vi "MAIN_call.vi"(8 "error IN":errorcluster, 11 "VISA resource name out":refnum<visa-resource-name>) -> (0 "error out":errorcluster)   [LabVIEW 2019]
uses:
  VI's/ESTADOS_ABS.ctl
  <vilib>/Utility/error.llb/Error Cluster From Error Code.vi
  <vilib>/ErrorRing/Error Ring.xnode
  SHARED VI'S/SHARED VI'S.lvlib
panel:
  in  "Tab Control":enum32{"Page 2"}(tab)
  in  "START":bool
  in  "home":bool
  in  "stop":bool
  in  "PARÁMETROS ENTRADA":T1={"mm en X"=308.5, "mm en Y"=455.0, "mm en Z"=0.0} {"mm en Z" min=0.0 max=40.0; "mm en Y" min=100.0 max=550.0; "mm en X" min=90.0 max=650.0}
  out "ESTADO ACTUAL":T2
  # "EXISTEN LIMITES DE SEGURIDAD PARA LOS CONTROLES  en mm X,Y,Z \nNO MODIFICARLOS!!"
  # "/* Teoricamente en X e Y:\n1mm= 91,32 pasos\n1cm = 913,2 pasos\n10 cm = 9132 pasos\n0.1 mm = 9,132 pasos aprox\n*/\nEl eje Z se mueve 1 mm por cada 3200 pulsos. Desde la ventosa hasta el tablero metalico hay aprox. 45mm (144000 pulsos teoricamente, NO PONER NUNCA ÉSTE VALOR )"
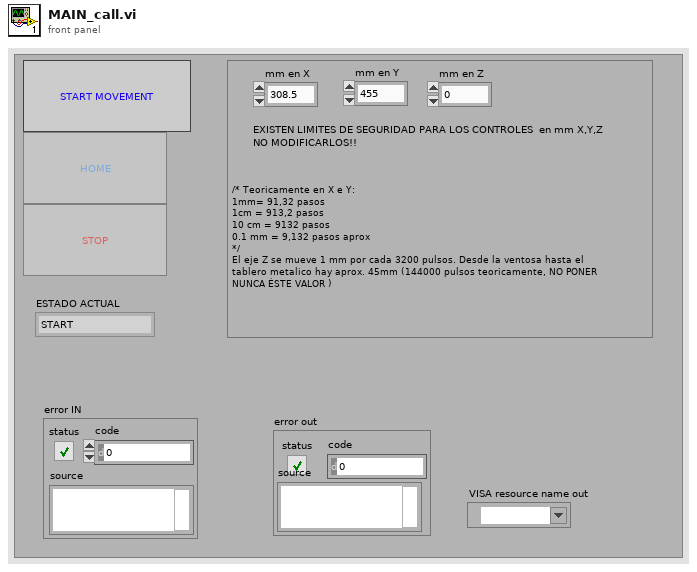
[diagram p1: front panel]
types:
  T1 = typedef "PARÁMETROS_ABSOLUTOS.ctl" = cluster{"mm en X":dbl, "mm en Y":dbl, "mm en Z":dbl}
  T2 = typedef "ESTADOS_ABS.ctl" = enum16{"START", "GESTION EVENTOS", "ENVIAR PARAMETROS", "HOME", "ERROR?", "SALIR"}
  T3 = enum8{"Enabled", "Disabled", "Disabled and Grayed Out"}
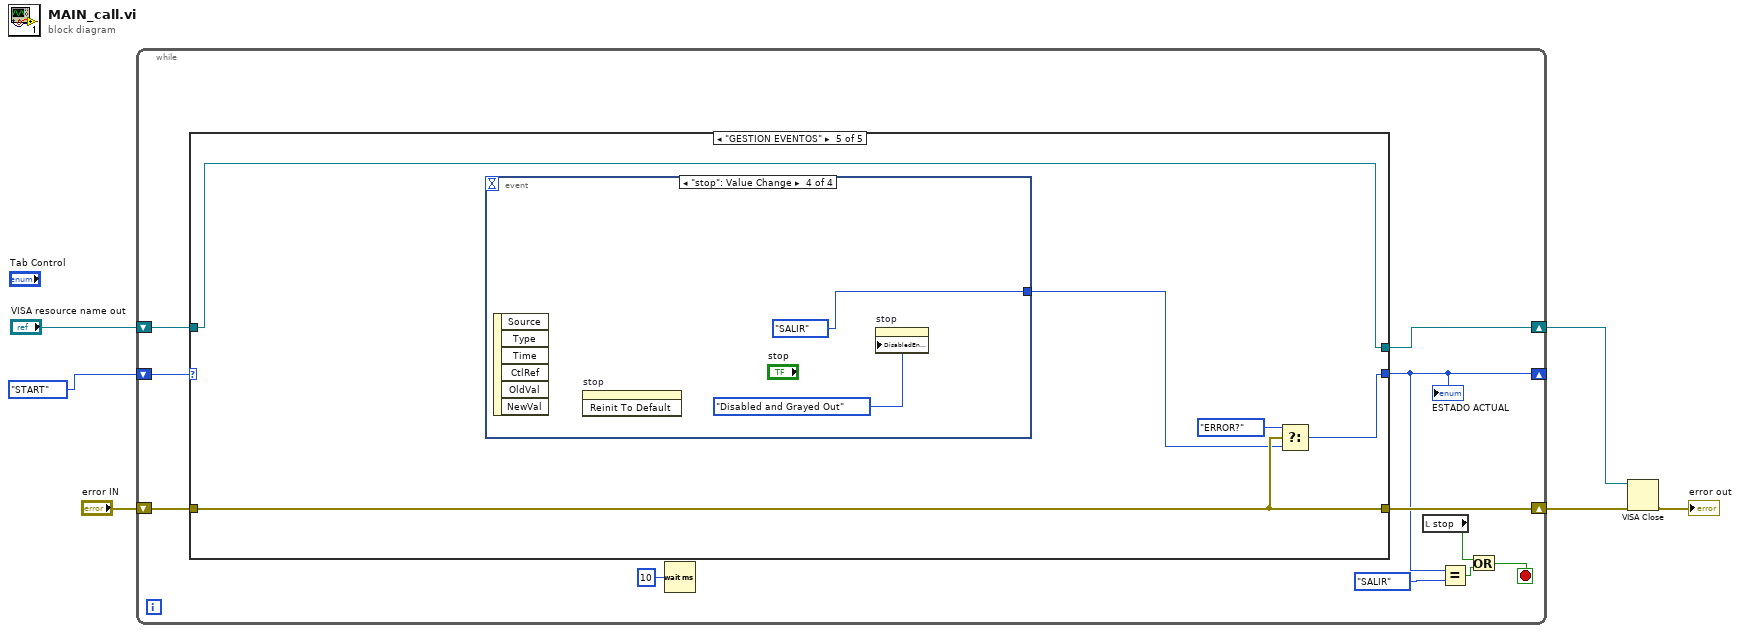
[diagram p0: block diagram]
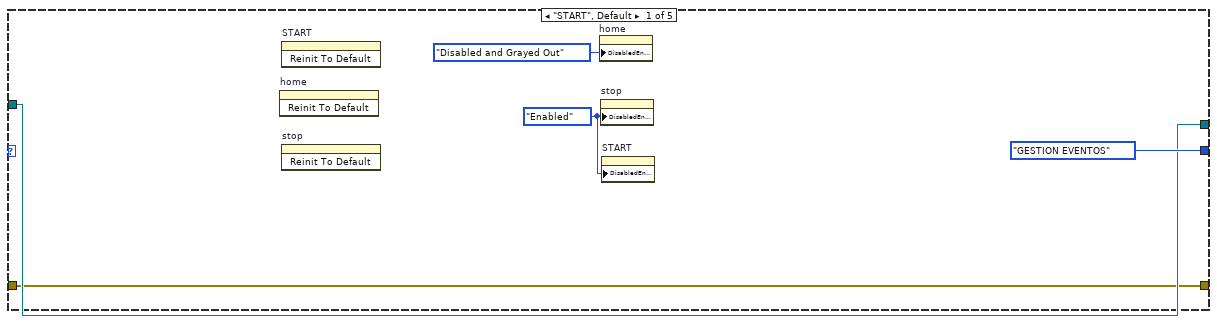
[diagram p2: hidden frame]
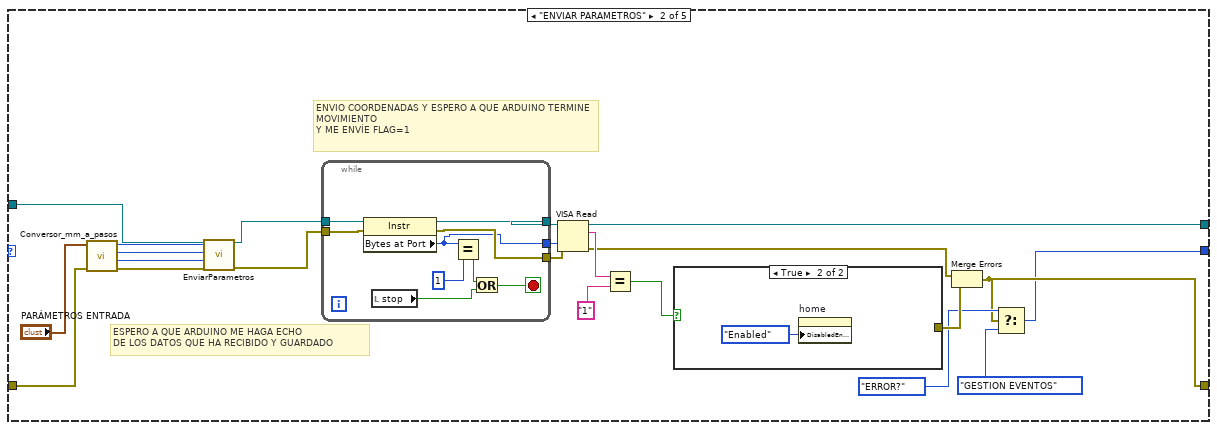
[diagram p3: hidden frame]
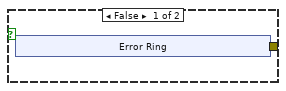
[diagram p4: hidden frame]
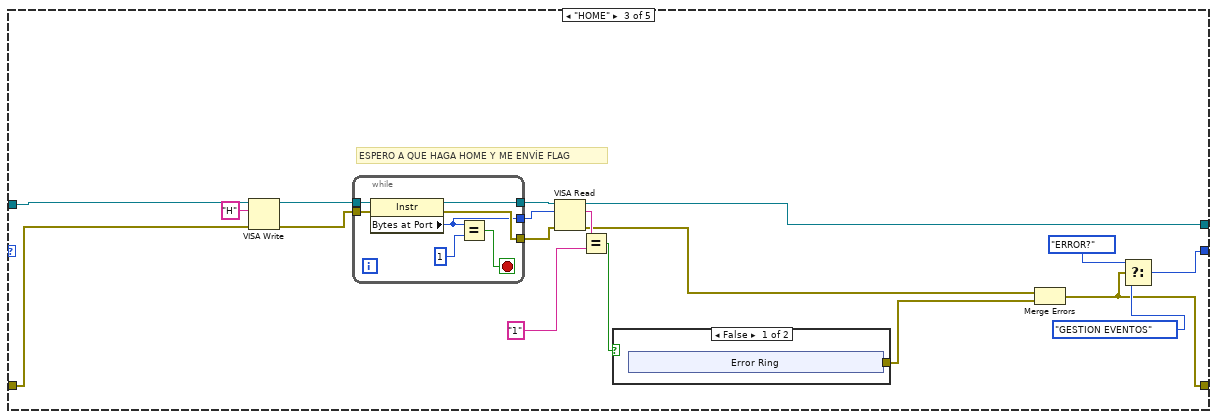
[diagram p5: hidden frame]
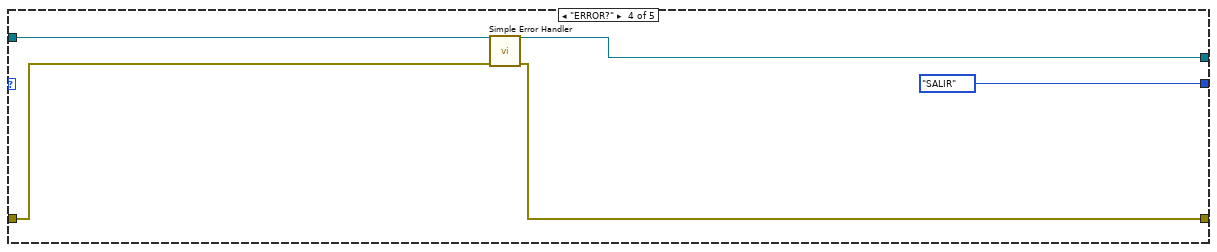
[diagram p7: hidden frame]
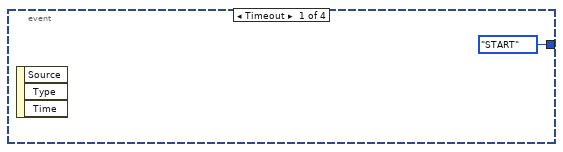
[diagram p8: hidden frame]
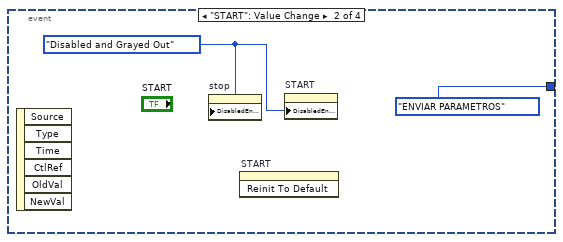
[diagram p9: hidden frame]
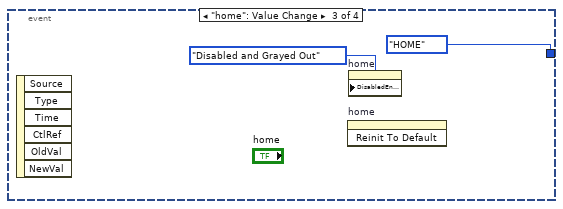
[diagram p10: hidden frame]
diagram:
  n1 = while {
    shift-right: [w10] -> _
    shift-left: ESTADOS_ABS."START" -> [w17]
    shift-right: [w12] -> w5
    shift-left: "error IN" -> [w16]
    shift-right: [w7] -> w3
    shift-left: "VISA resource name out" -> [w15]
    stop <- w13 stop-if-true
    n2 = case shown="\"GESTION EVENTOS\"" w17 {
      tunnel: [ESTADOS_ABS."GESTION EVENTOS" ("t") w33 w65 ESTADOS_ABS."SALIR" w98] -> w10
      tunnel: w16 -> [w20 w30 w77 w94 w97]
      tunnel: w15 -> [w21 w25 w78 w95 w100]
      tunnel: [w21 w40 w68 w95 w100] -> w7
      tunnel: [w20 w34 w62 w93 w97] -> w12
      frame "START", Default {
        w18 = T3."Enabled" ("Disabled")
        n3 = invoke on="home" class="Bool" method="Reinit To Default"() -> ()  [unwired: 3 in, 3 out]
        n4 = invoke on="START" class="Bool" method="Reinit To Default"() -> ()  [unwired: 3 in, 3 out]
        n5 = invoke on="stop" class="Bool (strict)" method="Reinit To Default"() -> ()  [unwired: 3 in, 3 out]
        n6 = property on="home" class="Bool"("DisabledEnum"=T3."Disabled and Grayed Out" ("Disabled")) -> ()  [unwired: 2 in, 2 out]
        n7 = property on="stop" class="Bool (strict)"("DisabledEnum"=w18) -> ()  [unwired: 2 in, 2 out]
        n8 = property on="START" class="Bool"("DisabledEnum"=w18) -> ()  [unwired: 2 in, 2 out]
      }
      frame "ENVIAR PARAMETROS" {
        # "ESPERO A QUE ARDUINO ME HAGA ECHO\nDE LOS DATOS QUE HA RECIBIDO Y GUARDADO"
        # "ENVIO COORDENADAS Y ESPERO A QUE ARDUINO TERMINE MOVIMIENTO\nY ME ENVÍE FLAG=1"
        n9 = call "Conversor_mm_a_pasos.vi"("error in (no error)"=w30, "PARÁMETROS ENTRADA"="PARÁMETROS ENTRADA") -> ("error out"=w26:errorcluster, "PASOS EN Z"=w27:i32, "PASOS EN Y"=w28:i32, "PASOS EN X"=w29:i32)  [unwired: 6 in]
        n10 = call "EnviarParametros.vi"("VISA resource name"=w25, "PASOS EN X"=w29, "PASOS EN Y"=w28, "PASOS EN Z"=w27, "error in (no error)"=w26) -> ("VISA resource name 2"=w24:refnum<visa-resource-name>, "error out"=w23:errorcluster)  [unwired: 9 in]
        n11 = while {
          tunnel: [w59] -> w43
          tunnel: [w58] -> w42
          tunnel: [w57] -> w32
          tunnel: w24 -> [w56]
          tunnel: w23 -> [w55]
          stop <- w53 stop-if-true
          n12 = property class="Instr"(reference=w56, error in=w55) -> (reference out=w59:refnum<visa-resource-name>, error out=w58:errorcluster, "Bytes at Port"=w57:u32)
          n13 = local read "stop"() -> (w52:bool)
          n14 = Equal?(x=w57, y=u32 1) -> (x = y?=w54:bool)
          n15 = Or(x=w54, y=w52) -> (x .or. y?=w53:bool)
        }
        n16 = VISA Read(VISA resource name=w43, byte count=w32, error in (no error)=w42) -> (VISA resource name out=w40:refnum<visa-resource-name>, read buffer=w41:string, error out=w38:errorcluster)  [unwired: 1 out]
        n17 = Equal?(x=w41, y="1") -> (x = y?=w39:bool)
        n18 = case shown="True" w39 {
          tunnel: [w45 _] -> w37
          frame False {
            n19 = xnode "Error Ring"() -> ("error out"=w45:errorcluster)
          }
          frame True {
            n20 = property on="home" class="Bool"("DisabledEnum"=T3."Enabled" ("Disabled")) -> ()  [unwired: 2 in, 2 out]
          }
        }
        n21 = Merge Errors(w38, w37) -> (w34:errorcluster)
        n22 = Select(t=ESTADOS_ABS."ERROR?", s=w34, f=ESTADOS_ABS."GESTION EVENTOS") -> (s? t:f=w33:T2)
      }
      frame "HOME" {
        # "ESPERO A QUE HAGA HOME Y ME ENVÍE FLAG"
        n23 = VISA Write(VISA resource name=w78, write buffer="H", error in (no error)=w77) -> (VISA resource name out=w69:refnum<visa-resource-name>, error out=w70:errorcluster)  [unwired: 1 out]
        n24 = while {
          tunnel: [w89] -> w75
          tunnel: [w88] -> w74
          tunnel: w70 -> [w87]
          tunnel: w69 -> [w86]
          tunnel: [w85] -> w63
          stop <- w91 stop-if-true
          n25 = property class="Instr"(reference=w86, error in=w87) -> (reference out=w89:refnum<visa-resource-name>, error out=w88:errorcluster, "Bytes at Port"=w85:u32)
          n26 = Equal?(x=w85, y=u32 1) -> (x = y?=w91:bool)
        }
        n27 = VISA Read(VISA resource name=w75, byte count=w63, error in (no error)=w74) -> (VISA resource name out=w68:refnum<visa-resource-name>, read buffer=w73:string, error out=w66:errorcluster)  [unwired: 1 out]
        n28 = Equal?(x=w73, y="1") -> (x = y?=w72:bool)
        n29 = case shown="False" w72 {
          tunnel: [w79 _] -> w67
          frame False {
            n30 = xnode "Error Ring"() -> ("error out"=w79:errorcluster)
          }
          frame True {
          }
        }
        n31 = Merge Errors(w66, w67) -> (w62:errorcluster)
        n32 = Select(t=ESTADOS_ABS."ERROR?", s=w62, f=ESTADOS_ABS."GESTION EVENTOS") -> (s? t:f=w65:T2)
      }
      frame "ERROR?" {
        n33 = call <vilib>:"Simple Error Handler.vi"("error in (no error)"=w94) -> ("error out"=w93:errorcluster)  [unwired: 4 in, 4 out]
      }
      frame "GESTION EVENTOS" {
        n34 = event shown="[3] \"stop\": Value Change" {
          selector: _ -> [_ _ _ _]
          dyn-events: _ -> [_ _ _ _]
          timeout: _ -> [_ _ _ _]
          tunnel: [ESTADOS_ABS."START" ("t") ESTADOS_ABS."ENVIAR PARAMETROS" ESTADOS_ABS."HOME" ("t") ESTADOS_ABS."SALIR" ("t")] -> w96
          event Timeout {
            n35 = event-data() -> ()  [unwired: 1 in, 3 out]
          }
          event "START": Value Change {
            w102 = T3."Disabled and Grayed Out" ("Disabled")
            n36 = event-data() -> ()  [unwired: 1 in, 6 out]
            n37 = property on="stop" class="Bool (strict)"("DisabledEnum"=w102) -> ()  [unwired: 2 in, 2 out]
            n38 = invoke on="START" class="Bool" method="Reinit To Default"() -> ()  [unwired: 3 in, 3 out]
            n39 = property on="START" class="Bool"("DisabledEnum"=w102) -> ()  [unwired: 2 in, 2 out]
          }
          event "home": Value Change {
            n40 = event-data() -> ()  [unwired: 1 in, 6 out]
            n41 = invoke on="home" class="Bool" method="Reinit To Default"() -> ()  [unwired: 3 in, 3 out]
            n42 = property on="home" class="Bool"("DisabledEnum"=T3."Disabled and Grayed Out" ("Disabled")) -> ()  [unwired: 2 in, 2 out]
          }
          event "stop": Value Change {
            n43 = event-data() -> ()  [unwired: 1 in, 6 out]
            n44 = invoke on="stop" class="Bool (strict)" method="Reinit To Default"() -> ()  [unwired: 3 in, 3 out]
            n45 = property on="stop" class="Bool (strict)"("DisabledEnum"=T3."Disabled and Grayed Out" ("Disabled")) -> ()  [unwired: 2 in, 2 out]
          }
        }
        n46 = Select(t=ESTADOS_ABS."ERROR?", s=w97, f=w96) -> (s? t:f=w98:T2)
      }
    }
    "ESTADO ACTUAL" <- w10
    n47 = Wait (ms)(milliseconds to wait=u32 10) -> ()  [unwired: 1 out]
    n48 = local read "stop"() -> (w8:bool)
    n49 = Equal?(x=w10, y=ESTADOS_ABS."SALIR") -> (x = y?=w11:bool)
    n50 = Or(x=w8, y=w11) -> (x .or. y?=w13:bool)
  }
  n51 = VISA Close(VISA resource name=w3, error in (no error)=w5) -> (error out=→"error out":errorcluster)
